vi "RR_OneCh_MovAvg.vi"(1 "SampleSize":u8=6, 3 "DataIN":dbl) -> (0 "Mean":dbl format="%0.2f")   [LabVIEW 2017]
doc: "Moving Average VI to compute the specified sample base moving average. \n\nR Raghunathan.\n01 April 2016"
uses:
  <vilib>/Analysis/baseanly.llb/Mean (DBL).vi
  <vilib>/Analysis/NI_AALBase.lvlib
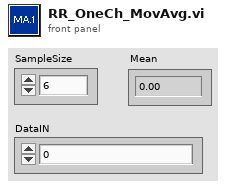
[diagram p1: front panel]
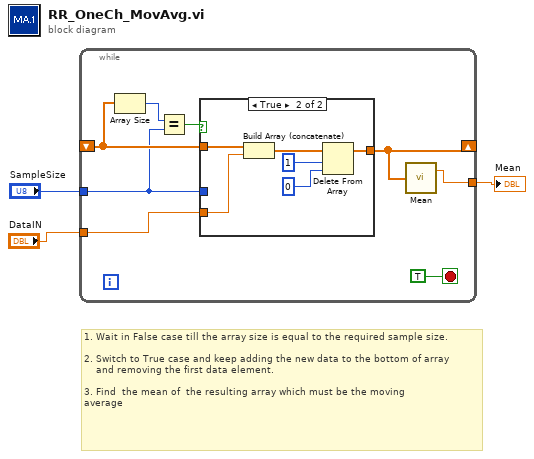
[diagram p0: block diagram]
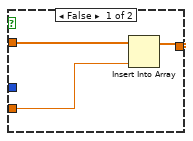
[diagram p2: hidden frame]
diagram:
  # "1. Wait in False case till the array size is equal to the required sample size.\n\n2. Switch to True case and keep adding the new data to the bottom of array \n    and removing the first data element. \n\n3. Find  the mean of  the resulting array which must be the moving \naverage"
  n1 = while {
    shift-right: [w7] -> _
    shift-left: _ -> [w10]
    tunnel: "SampleSize" -> [w6]
    tunnel: "DataIN" -> [w5]
    tunnel: [w4] -> w3
    stop <- TRUE stop-if-true
    n2 = Array Size(array=w10) -> (size(s)=w9:i32)
    n3 = Equal?(x=w9, y=w6) -> (x = y?=w8:bool)
    n4 = case shown="True" w8 {
      tunnel: [w14 w19] -> w7
      tunnel: w10 -> [w13 w15]
      tunnel: w5 -> [w12 w16]
      tunnel: w6 -> [_ _]
      frame False {
        n5 = Insert Into Array(array=w13, new element=w12) -> (w14:dbl[])  [unwired: 1 in]
      }
      frame True {
        n6 = Build Array (concatenate)(w15, w16) -> (w20:dbl[])
        n7 = Delete From Array(array=w20, length=1, index=0) -> (array with subset deleted=w19:dbl[])  [unwired: 1 out]
      }
    }
    n8 = call-poly <vilib>:"Mean.vi"("X"=w7) -> ("mean"=w4:dbl)  [unwired: 1 out]
  }
  "Mean" <- w3
